vi "Delete From Array.vi"(3 "error in (no error)":errorcluster, 4 "index (last elem)":i32=-1, 5 "Controller Array in":refnum<class "Controller Array.lvclass">) -> (0 "error out":errorcluster, 1 "deleted portion":refnum<class "Generic Plugin.lvclass">, 2 "Controller Array out":refnum<class "Controller Array.lvclass">)   [LabVIEW 2020, in "RxnRover.lvlib" / "Controller Array.lvclass"]
doc: "Deletes a controller entry from the array, returning the deleted item."
uses:
  Controller Array.lvclass
  Controller/Generic Plugin.lvclass
  Controller Array.lvclass/Controller Array.ctl
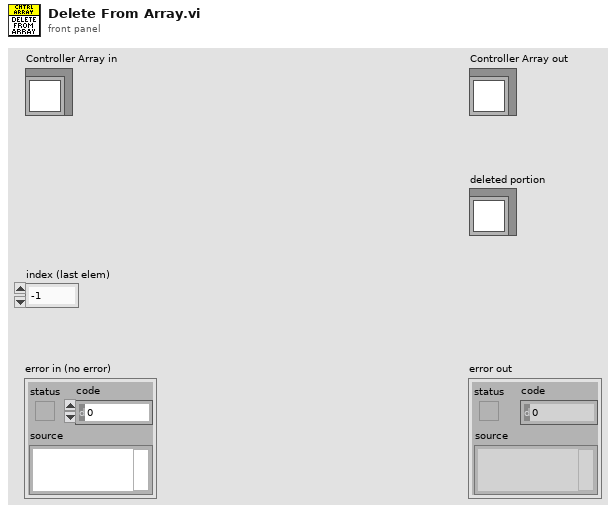
[diagram p1: front panel]
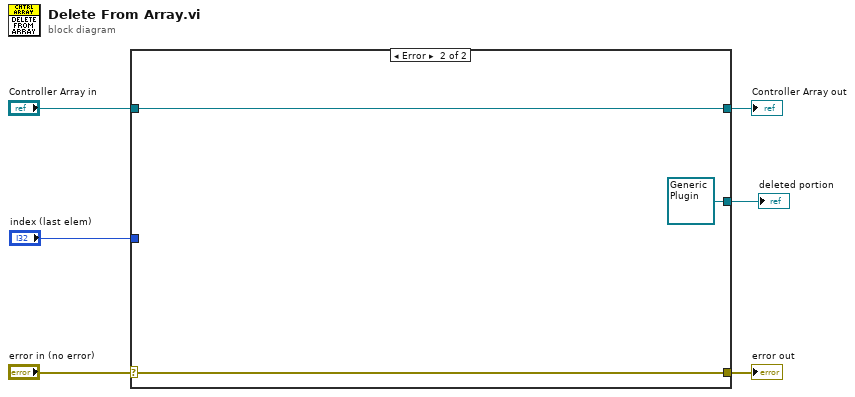
[diagram p0: block diagram]
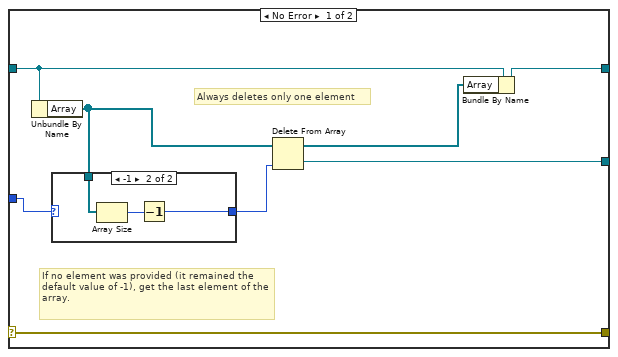
[diagram p2: hidden frame]
diagram:
  n1 = case shown="Error" "error in (no error)" {
    selector: "error in (no error)" -> [w14 w21]
    tunnel: [w14 w21] -> w5
    tunnel: [w13 w20] -> w3
    tunnel: "Controller Array in" -> [w11 w20]
    tunnel: "index (last elem)" -> [w10 _]
    tunnel: [w7 refnum<class "Generic Plugin.lvclass"> refnum ("Controller.lvclass")] -> w1
    frame No Error {
      # "Always deletes only one element"
      # "If no element was provided (it remained the default value of -1), get the last element of the array."
      n2 = Unbundle By Name(w11) -> ("Array"=w9:refnum<class "Generic Plugin.lvclass">[])
      n3 = case shown="-1" w10 {
        selector: w10 -> [w15 _]
        tunnel: w9 -> [_ w18]
        tunnel: [w15 w16] -> w8
        frame Default {
        }
        frame -1 {
          n4 = Array Size(array=w18) -> (size(s)=w17:i32)
          n5 = Decrement(x=w17) -> (x-1=w16:i32)
        }
      }
      n6 = Delete From Array(array=w9, index=w8) -> (deleted portion=w7:refnum<class "Generic Plugin.lvclass">, array with subset deleted=w12:refnum<class "Generic Plugin.lvclass">[])  [unwired: 1 in]
      n7 = Bundle By Name(cluster=w11, "Array"=w12) -> (w13:refnum<class "Controller Array.lvclass">)
    }
    frame Error {
    }
  }
  "error out" <- w5
  "Controller Array out" <- w3
  "deleted portion" <- w1
